vi "Get Column Config.vi"(8 "error in (no error)":errorcluster, 11 "Table Configuration in":refnum<class "Table Configuration.lvclass">) -> (0 "error out":errorcluster, 2 "Column Configuration":refnum<class "Column Configuration.lvclass">, 3 "Table Configuration out":refnum<class "Table Configuration.lvclass">)   [LabVIEW 2020, in "Table.lvlib" / "Table Configuration.lvclass"]
uses:
  Table Configuration.lvclass
  Column Interface/Column Configuration Interface Class/Column Configuration.lvclass
  Table Configuration.lvclass/Table Configuration.ctl
  Basic Columns/Basic Column Configuration/Basic Column Configuration.lvclass
  C:/Users/User/Desktop/Raman Program/Database OOP/source/Database OOP/Column Interface/Column Configuration Interface Class/Column Configuration.lvclass
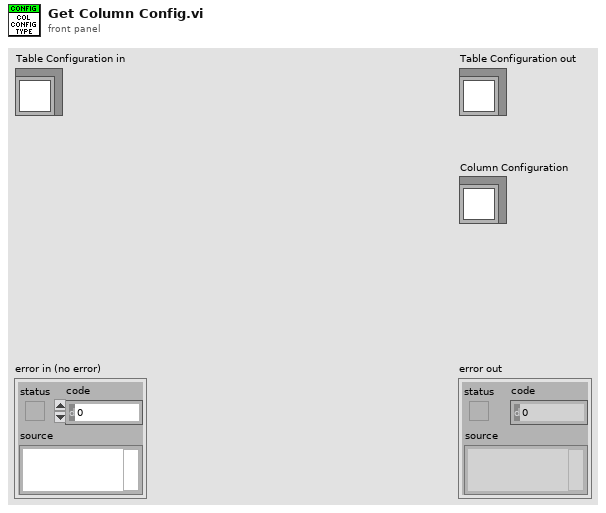
[diagram p1: front panel]
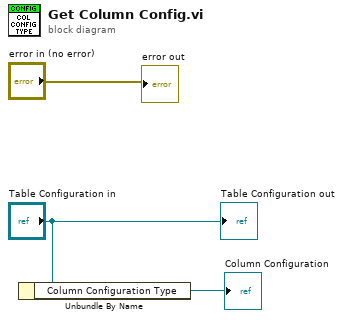
[diagram p0: block diagram]
diagram:
  n1 = Unbundle By Name("Table Configuration in") -> ("Column Configuration Type"=→"Column Configuration":refnum<class "Basic Column Configuration.lvclass">)
  "error out" <- "error in (no error)"
  "Table Configuration out" <- "Table Configuration in"
